vi "IMS Stepper Read Velocity.vi"(4 "error in (no error)":errorcluster, 7 "Instrument Address":refnum<visa-resource-name>) -> (0 "error out":errorcluster, 2 "Velocity":i32, 3 "dup VISA Resource Name":refnum<visa-resource-name>)   [LabVIEW 2020]
uses:
  <vilib>/regexp/Match Regular Expression.xnode
panel:
  out "Response":string
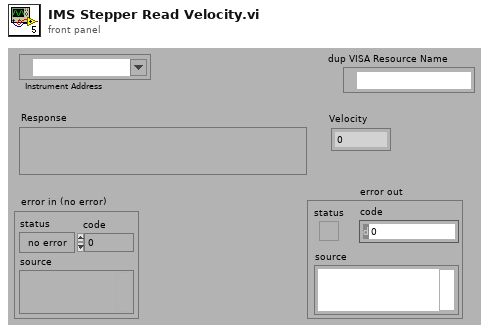
[diagram p1: front panel]
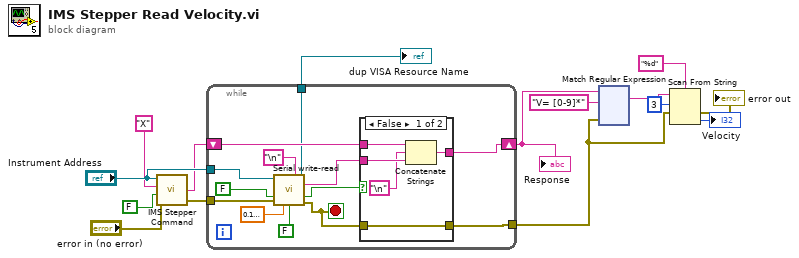
[diagram p0: block diagram]
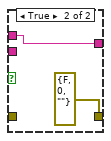
[diagram p2: hidden frame]
diagram:
  n1 = call "IMS Stepper Command.vi"("Instrument Address"="Instrument Address", "Command"="X", "Mode"=FALSE, "error in (no error)"="error in (no error)") -> ("Response"=w13:string, "error out"=w14:errorcluster)  [unwired: 2 in, 1 out]
  n2 = while {
    tunnel: "Instrument Address" -> [w28]
    tunnel: w14 -> [w27]
    shift-right: [w20] -> w12
    shift-left: w13 -> [w22]
    tunnel: [w17] -> w1
    tunnel: [w18] -> w2
    stop <- w16 stop-if-true
    n3 = call "Serial write-read.vi"("VISA Resource Name"=w28, "EOT Chars (cr/lf)"="\n", "Clear Buffer?"=FALSE, "error in (no error)"=w27, "Timeout Limit"=sgl 0.1, "Read Echo?"=FALSE) -> ("dup VISA Resource Name"=w18:refnum<visa-resource-name>, "Serial Read"=w21:string, "Timeout"=w19:bool, "error out"=w16:errorcluster)  [unwired: 4 in, 2 out]
    n4 = case shown="False" w19 {
      tunnel: w22 -> [w33 w35]
      tunnel: w21 -> [w31 _]
      tunnel: [w32 w35] -> w20
      tunnel: [w29 errorcluster {"status"=FALSE, "code"=0, "source"=""} ("error out")] -> w17
      tunnel: w16 -> [w29 _]
      frame False {
        n5 = Concatenate Strings(w33, "\n", w31) -> (w32:string)
      }
      frame True {
      }
    }
  }
  "Response" <- w12
  "dup VISA Resource Name" <- w2
  n6 = xnode "Match Regular Expression"("input string"=w12, "regular expression"="V= [0-9]*", "error in"=w1) -> ("whole match"=w10:string)  [unwired: 3 in, 4 out]
  n7 = Scan From String(format string="%d", input string=w10, initial scan location=u32 3, error in=w1) -> (error out=→"error out":errorcluster, output 1=→"Velocity":i32)  [unwired: 1 in, 2 out]
